vi "RobotIsConnected.vi"(2 "robot":refnum<k24>, 3 "error in":errorcluster) -> (0 "Connected":bool, 1 "error out":errorcluster)   [LabVIEW 2018, in "UnderAutomation.Fanuc.lvlib"]
uses:
  UnderAutomation.Fanuc.lvlib
  C:/Users/fg/Documents/Fanuc.vi/LabVIEW_2024/UnderAutomation.Fanuc/lib/UnderAutomation.Fanuc.dll
  LabVIEW_2024/UnderAutomation.Fanuc/lib/UnderAutomation.Fanuc.dll
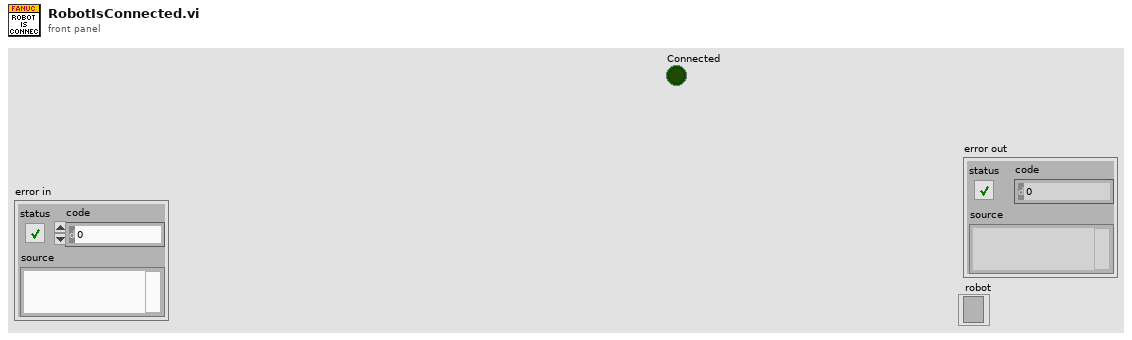
[diagram p1: front panel]
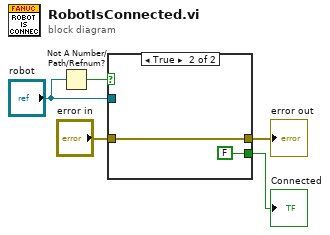
[diagram p0: block diagram]
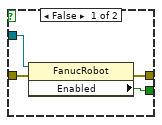
[diagram p2: hidden frame]
diagram:
  n1 = Not A Number/Path/Refnum?(number/path/refnum="robot") -> (NaN/Path/Refnum?=w1:bool)
  n2 = case shown="True" w1 {
    tunnel: [w9 FALSE ("Enabled")] -> w5
    tunnel: [w8 w11] -> w4
    tunnel: "error in" -> [w7 w11]
    tunnel: "robot" -> [w6 _]
    frame False {
      n3 = property class="FanucRobot"(reference=w6, error in=w7) -> (error out=w8:errorcluster, "Enabled"=w9:bool)  [unwired: 1 out]
    }
    frame True {
    }
  }
  "error out" <- w4
  "Connected" <- w5
